vi "Save DUT Information.vi"(8 "error in (no error)":errorcluster, 10 "DUT Info":T1, 11 "csv-formatter in":refnum<class "csv-formatter.lvclass">) -> (0 "error out":errorcluster, 3 "csv-formatter out":refnum<class "csv-formatter.lvclass">)   [LabVIEW 2015, in "csv-formatter.lvclass"]
doc: "This VI will save the DUT Information to the permanent report"
uses:
  csv-formatter.lvclass
  Report Information/DUT Information.ctl
  csv-formatter.lvclass/csv-formatter.ctl
  <vilib>/Utility/file.llb/Read Delimited Spreadsheet (string).vi
  <vilib>/Utility/file.llb/Write Delimited Spreadsheet (string).vi
  Report Information/Report Information.lvclass
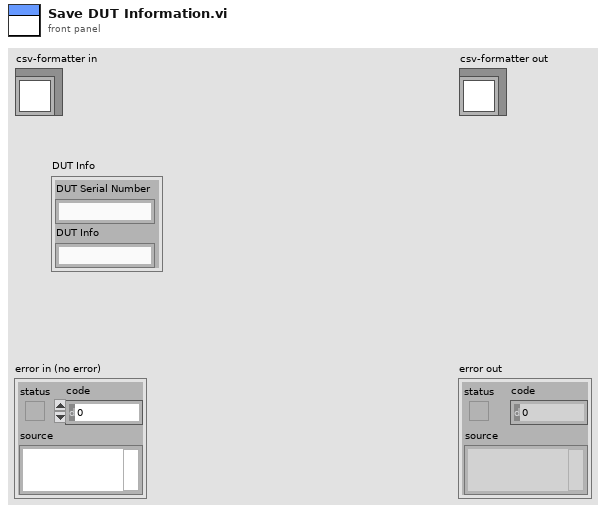
[diagram p1: front panel]
types:
  T1 = typedef "Report Information.lvclass/DUT Information.ctl" = cluster{"DUT Serial Number":string, "DUT Info":string}
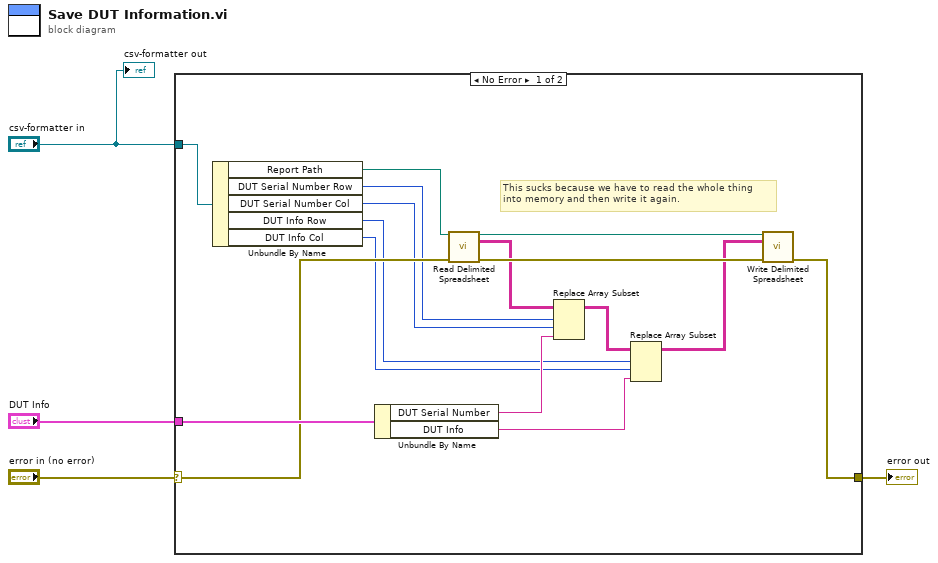
[diagram p0: block diagram]
diagram:
  n1 = case shown="No Error" "error in (no error)" {
    selector: "error in (no error)" -> [w16 w21]
    tunnel: "DUT Info" -> [w18 _]
    tunnel: "csv-formatter in" -> [w17 _]
    tunnel: [w14 w21] -> w1
    frame No Error {
      # "This sucks because we have to read the whole thing\ninto memory and then write it again."
      n2 = Unbundle By Name(w17) -> ("Report Path"=w20:path, "DUT Serial Number Row"=w8:i32, "DUT Serial Number Col"=w7:i32, "DUT Info Row"=w6:i32, "DUT Info Col"=w5:i32)
      n3 = Unbundle By Name(w18) -> ("DUT Serial Number"=w9:string, "DUT Info"=w10:string)
      n4 = call-poly <vilib>:"Read Delimited Spreadsheet.vi"("file path (dialog if empty)"=w20, "error in (no error)"=w16) -> ("new file path (Not A Path if cancelled)"=w19:path, "all rows"=w13:string[][], "error out"=w15:errorcluster)  [unwired: 8 in, 3 out]
      n5 = Replace Array Subset(array=w13, new element=w9, index (row)=w8, index (col)=w7) -> (w12:string[][])
      n6 = Replace Array Subset(array=w12, new element=w10, index (row)=w6, index (col)=w5) -> (w11:string[][])
      n7 = call-poly <vilib>:"Write Delimited Spreadsheet.vi"("file path (dialog if empty)"=w19, "2D data"=w11, "error in (no error)"=w15) -> ("error out"=w14:errorcluster)  [unwired: 11 in, 1 out]
    }
    frame Error {
    }
  }
  "error out" <- w1
  "csv-formatter out" <- "csv-formatter in"
